vi "Write Module Decimation.vi"(7 "Module ID":string, 8 "error in":errorcluster, 10 "Module Decimation":T1={"Decimation"=1, "Offset"=0}, 11 "Standard Engine Repo Data in":refnum<class "Standard Engine Configuration.lvclass">) -> (0 "error out":errorcluster, 3 "Standard Engine Repo Data out":refnum<class "Standard Engine Configuration.lvclass">)   [LabVIEW 2013, in "Standard Engine Configuration.lvclass"]
uses:
  Standard Engine Configuration.lvclass
  Module Decimation.ctl
  Standard Engine Configuration.lvclass/Standard Engine Configuration.ctl
  <vilib>/NI/Configuration Framework/NISE_CEF_TreeControl.lvlib
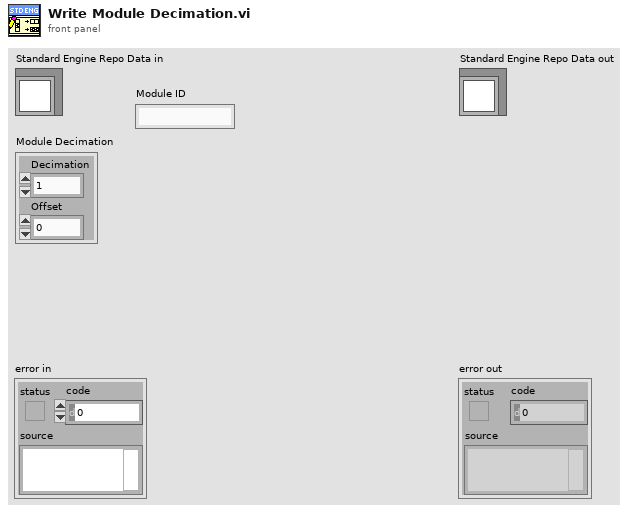
[diagram p1: front panel]
types:
  T1 = typedef "Standard Engine Configuration.lvclass/Module Decimation.ctl" = cluster{"Decimation":u16, "Offset":u16}
  T2 = typedef "Standard Engine Configuration.lvclass/Module Specific Configuration.ctl" = cluster{"Module ID":string, "Module Decimation":T1, "Module Error Configuration":T3, "execution order priority":i32, "async?":bool, "error tag":string}
  T3 = typedef "Standard Engine Configuration.lvclass/Module Error Configuration.ctl" = cluster{"Module Error Configuration":T4[]}
  T4 = typedef "Standard Engine Configuration.lvclass/Error Actions By Category.ctl" = cluster{"error classification":T5, "Error Actions":T6[]}
  T5 = typedef "TBM module execution interface.lvclass/error classification.ctl" = enum16{"unknown", "none", "trivial", "recoverable", "critical"}
  T6 = typedef "Standard Engine Configuration.lvclass/Error Actions.ctl" = enum16{"Clear", "Notify", "Stop Component", "Stop Engine", "Safe State", "Attempt Recovery"}
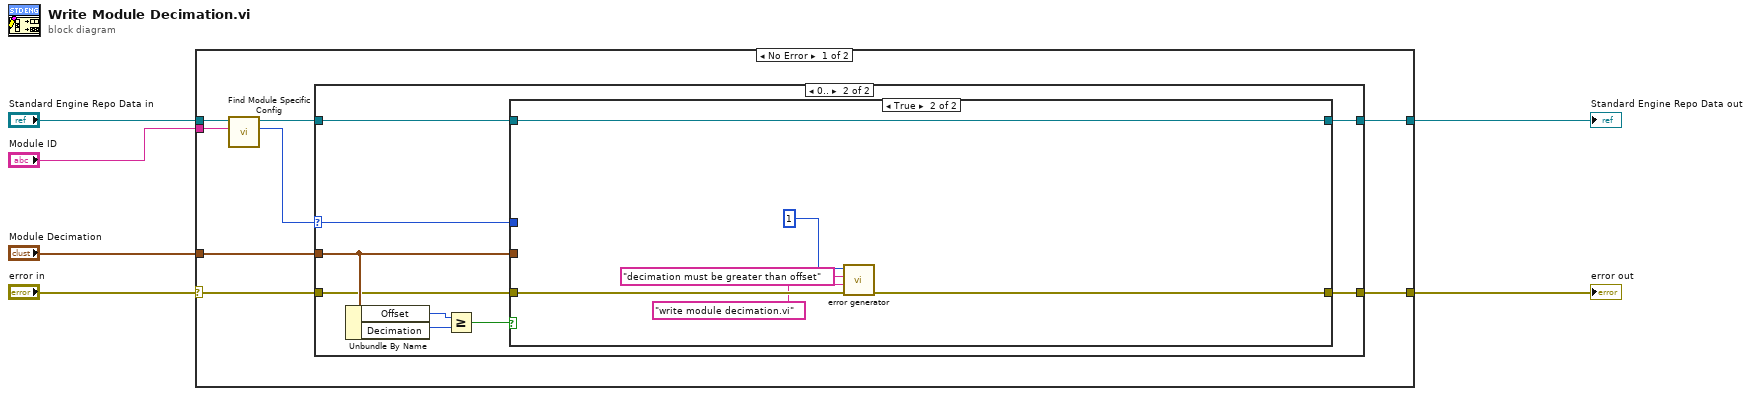
[diagram p0: block diagram]
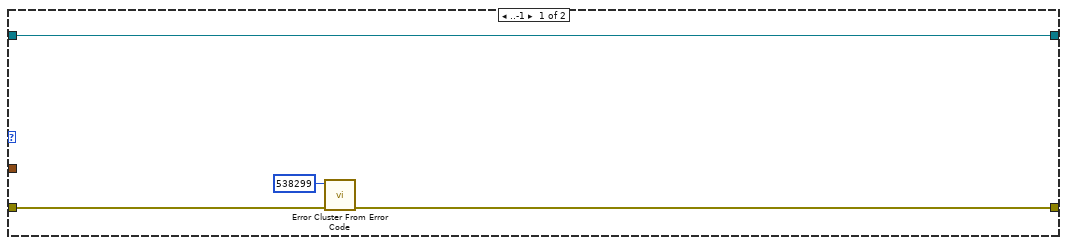
[diagram p2: hidden frame]
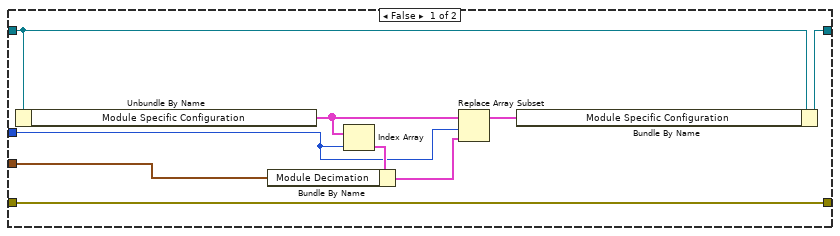
[diagram p3: hidden frame]
diagram:
  n1 = case shown="No Error" "error in" {
    selector: "error in" -> [w10 w44]
    tunnel: "Standard Engine Repo Data in" -> [w14 w43]
    tunnel: "Module ID" -> [w13 _]
    tunnel: [w8 w43] -> w1
    tunnel: [w9 w44] -> w2
    tunnel: "Module Decimation" -> [w7 _]
    frame No Error {
      n2 = call "Find Module Specific Config.vi"("Module ID"=w13, "Standard Engine Repo Data in"=w14) -> ("Index"=w11:i32, "Standard Engine Repo Data out"=w12:refnum<class "Standard Engine Configuration.lvclass">)  [unwired: 8 in]
      n3 = case shown="0.." w11 {
        selector: w11 -> [_ w27]
        tunnel: w12 -> [w17 w26]
        tunnel: w10 -> [w18 w19]
        tunnel: [w16 w20] -> w9
        tunnel: [w17 w25] -> w8
        tunnel: w7 -> [_ w24]
        frame ..-1 {
          n4 = call <vilib>:"Error Cluster From Error Code.vi"("error in (no error)"=w18, "error code (0)"=538299) -> ("error out"=w16:errorcluster)  [unwired: 7 in]
        }
        frame 0.. {
          n5 = Unbundle By Name(w24) -> ("Offset"=w23:u16, "Decimation"=w22:u16)
          n6 = Greater Or Equal?(x=w23, y=w22) -> (x >= y?=w21:bool)
          n7 = case shown="True" w21 {
            tunnel: w27 -> [w35 _]
            tunnel: w26 -> [w32 w42]
            tunnel: [w30 w42] -> w25
            tunnel: w24 -> [w29 _]
            tunnel: [w28 w40] -> w20
            tunnel: w19 -> [w28 w41]
            frame False {
              n8 = Unbundle By Name(w32) -> ("Module Specific Configuration"=w34:T2[])
              n9 = Index Array(array=w34, index=w35) -> (element=w36:T2)
              n10 = Bundle By Name(cluster=w36, "Module Decimation"=w29) -> (w33:T2)
              n11 = Replace Array Subset(array=w34, new element=w33, index=w35) -> (w31:T2[])
              n12 = Bundle By Name(cluster=w32, "Module Specific Configuration"=w31) -> (w30:refnum<class "Standard Engine Configuration.lvclass">)
            }
            frame True {
              n13 = call <vilib>:"error generator.vi"("error in"=w41, "source"="write module decimation.vi", "append error message"="decimation must be greater than offset", "error code (0)"=1) -> ("error out"=w40:errorcluster)  [unwired: 5 in]
            }
          }
        }
      }
    }
    frame Error {
    }
  }
  "error out" <- w2
  "Standard Engine Repo Data out" <- w1
